vi "VI Reference To IWin32Window Reference.vi"(8 "error in (no error)":errorcluster, 11 "VI Reference":refnum<vi>) -> (0 "error out":errorcluster, 3 "System.Windows.Forms.IWin32Window":refnum<k24>)   [LabVIEW 2020]
doc: "This VI obtains a IWin32Window Reference for the VI Front Panel that is specified by the VI Reference."
uses:
  System.Windows.Forms
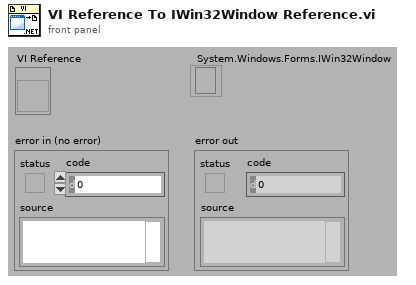
[diagram p1: front panel]
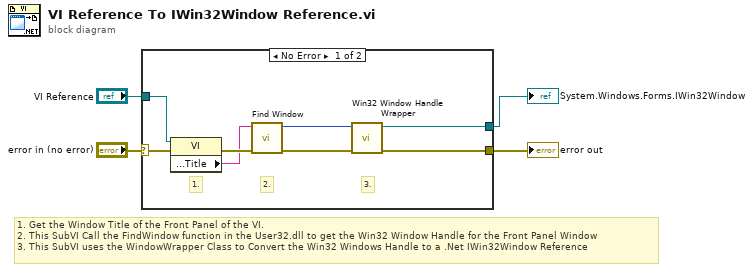
[diagram p0: block diagram]
diagram:
  # "1. Get the Window Title of the Front Panel of the VI.\n2. This SubVI Call the FindWindow function in the User32.dll to get the Win32 Window Handle for the Front Panel Window\n3. This SubVI uses the WindowWrapper Class to Convert the Win32 Windows Handle to a .Net IWin32Window Reference"
  n1 = case shown="No Error" "error in (no error)" {
    selector: "error in (no error)" -> [w6 w13]
    tunnel: "VI Reference" -> [w8 _]
    tunnel: [w7 w13] -> w3
    tunnel: [w5 _] -> w1
    frame No Error {
      # "3."
      # "2."
      # "1."
      n2 = property class="VI"(reference=w8, error in=w6) -> (error out=w10:errorcluster, "Front Panel.Title"=w9:string)  [unwired: 1 out]
      n3 = call "Find Window.vi"("error in (no error)"=w10, "Window Name"=w9) -> ("error out"=w12:errorcluster, "Win32 Window Handle"=w11:i32)  [unwired: 8 out]
      n4 = call "Win32 Window Handle Wrapper.vi"("error in (no error)"=w12, "Win32 Window Handle"=w11) -> ("error out"=w7:errorcluster, "System.Windows.Forms.IWin32Window"=w5:refnum<k24>)  [unwired: 2 in, 6 out]
    }
    frame Error {
    }
  }
  "System.Windows.Forms.IWin32Window" <- w1
  "error out" <- w3
